vi "Find Observer by Name.vi"(8 "error in (no error)":errorcluster, 10 "Observer Name":string, 11 "Vessel in":refnum<class "Vessel.lvclass">) -> (0 "error out":errorcluster, 2 "Index":i32, 3 "Vessel out":refnum<class "Vessel.lvclass">)   [LabVIEW 2014, in "Vessel.lvclass"]
uses:
  Vessel.lvclass
  Vessel.lvclass/Vessel.ctl
  Observer/Observer.lvclass
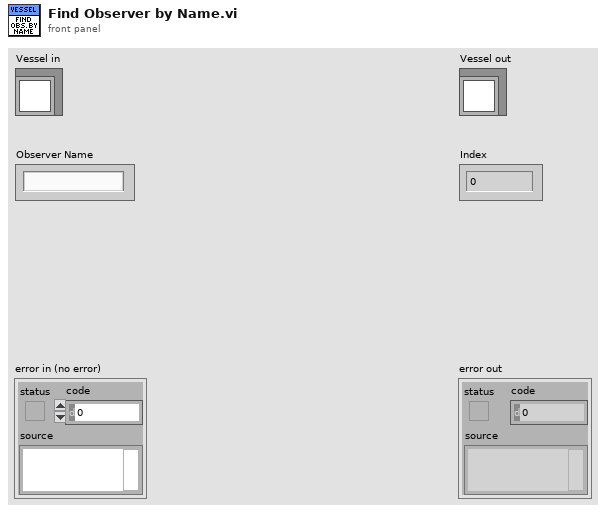
[diagram p1: front panel]
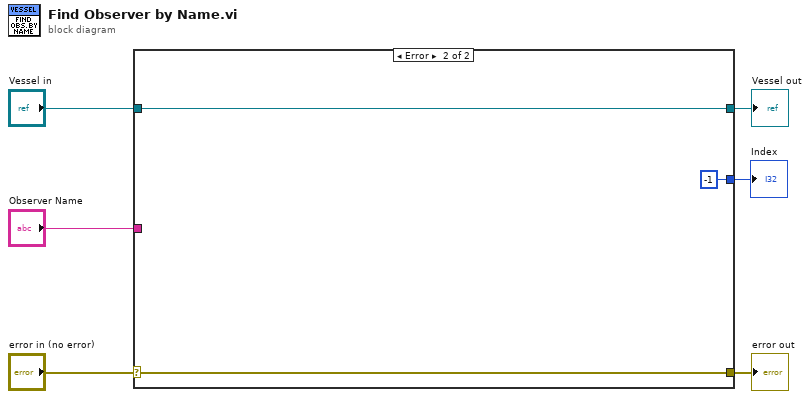
[diagram p0: block diagram]
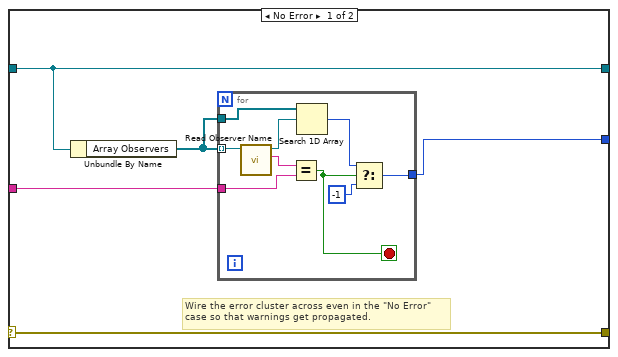
[diagram p2: hidden frame]
diagram:
  n1 = case shown="Error" "error in (no error)" {
    selector: "error in (no error)" -> [w11 w23]
    tunnel: [w11 w23] -> w5
    tunnel: [w10 w22] -> w3
    tunnel: "Vessel in" -> [w10 w22]
    tunnel: "Observer Name" -> [w8 _]
    tunnel: [w7 -1 ("index of element")] -> w1
    frame No Error {
      # "Wire the error cluster across even in the \"No Error\"\ncase so that warnings get propagated."
      n2 = Unbundle By Name(w10) -> ("Array Observers"=w9:refnum<class "Observer.lvclass">[])
      n3 = for {
        tunnel: w9 -> [w20] mode=indexing
        tunnel: w9 -> [w19]
        tunnel: w8 -> [w16]
        tunnel: [w14] -> w7
        stop <- w13 stop-if-true
        n4 = call-dynamic "Read Observer Name.vi"("Observer in"=w20) -> ("Observer Name"=w17:string, "Observer out"=w18:refnum<class "Observer.lvclass">)  [unwired: 8 in, 1 out]
        n5 = Equal?(x=w17, y=w16) -> (x = y?=w13:bool)
        n6 = Search 1D Array(1D array=w19, element=w18) -> (index of element=w15:i32)  [unwired: 1 in]
        n7 = Select(t=w15, s=w13, f=-1) -> (s? t:f=w14:i32)
      }
    }
    frame Error {
    }
  }
  "error out" <- w5
  "Vessel out" <- w3
  "Index" <- w1
